vi "Daten am cRIO Speichern.vi"(6 "Aktionen":T1, 10 "gespeichert":bool) -> (2 "gespeichert":bool, 3 "speichern":bool)   [LabVIEW 2020, in "allgemeine Sub-VIs.lvlib"]
uses:
  allgemeine Sub-VIs.lvlib
  Aktionen Daten am cRIO speichern.ctl
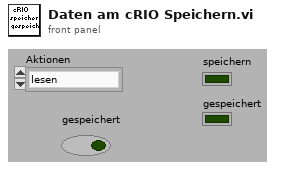
[diagram p1: front panel]
types:
  T1 = typedef "allgemeine Sub-VIs.lvlib/Aktionen Daten am cRIO speichern.ctl" = enum16{"lesen", "speichern setzen", "speichern reset", "gespeichert"}
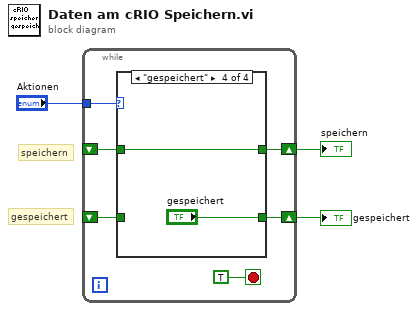
[diagram p0: block diagram]
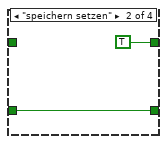
[diagram p3: hidden frame]
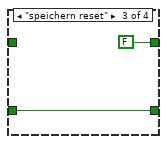
[diagram p4: hidden frame]
diagram:
  # "gespeichert"
  # "speichern"
  n1 = while {
    shift-right: [w8] -> w2
    shift-left: _ -> [w6]
    tunnel: "Aktionen" -> [w9]
    shift-right: [w7] -> w1
    shift-left: _ -> [w5]
    stop <- TRUE stop-if-true
    n2 = case shown="\"gespeichert\"" w9 {
      tunnel: [w11 TRUE ("speichern") FALSE ("speichern") w17] -> w8
      tunnel: [w10 w12 w14 "gespeichert"] -> w7
      tunnel: w6 -> [w11 _ _ w17]
      tunnel: w5 -> [w10 w12 w14 _]
      frame "lesen", Default {
      }
      frame "speichern setzen" {
      }
      frame "speichern reset" {
      }
      frame "gespeichert" {
      }
    }
  }
  "speichern" <- w2
  "gespeichert" <- w1
